vi "Request Data JSON.vi"(8 "error in (no error)":errorcluster, 11 "SetCurrentProfile in":refnum<class "SetCurrentProfile.lvclass">) -> (0 "error out":errorcluster, 2 "Request Data JSON":string, 3 "SetCurrentProfile out":refnum<class "SetCurrentProfile.lvclass">)   [LabVIEW 2022 SP3, in "obs-websocket-lv.lvlib" / "SetCurrentProfile.lvclass"]
uses:
  SetCurrentProfile.lvclass
  SetCurrentProfile.lvclass/SetCurrentProfile.ctl
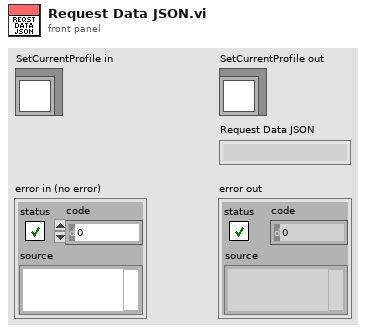
[diagram p1: front panel]
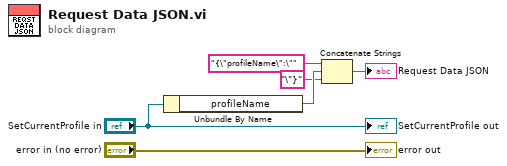
[diagram p0: block diagram]
diagram:
  n1 = Unbundle By Name("SetCurrentProfile in") -> ("profileName"=w4:string)
  n2 = Concatenate Strings("{\"profileName\":\"" ("string"), w4, "\"}" ("string")) -> (→"Request Data JSON":string)
  "error out" <- "error in (no error)"
  "SetCurrentProfile out" <- "SetCurrentProfile in"
